vi "GetNetworkTime.vi"(8 "error in (no error)":errorcluster, 11 "NetworkPlugin in":refnum<class "NetworkPlugin.lvclass">) -> (0 "error out":errorcluster, 3 "NetworkPlugin out":refnum<class "NetworkPlugin.lvclass">)   [LabVIEW 2014, in "NetworkImpairmentPlugins.lvlib" / "NetworkPlugin.lvclass"]
uses:
  NetworkPlugin.lvclass
  NetworkImpairmentPluginBase_class/Accessors/Read TimeArray.vi
  NetworkImpairmentPluginBase_class/Accessors/Read NetImpParams.vi
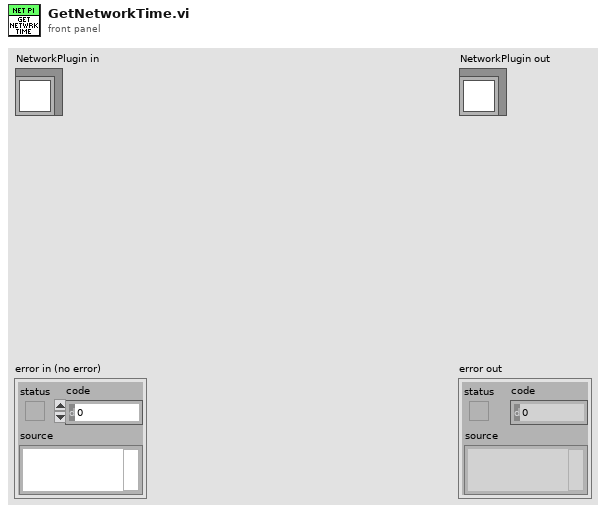
[diagram p1: front panel]
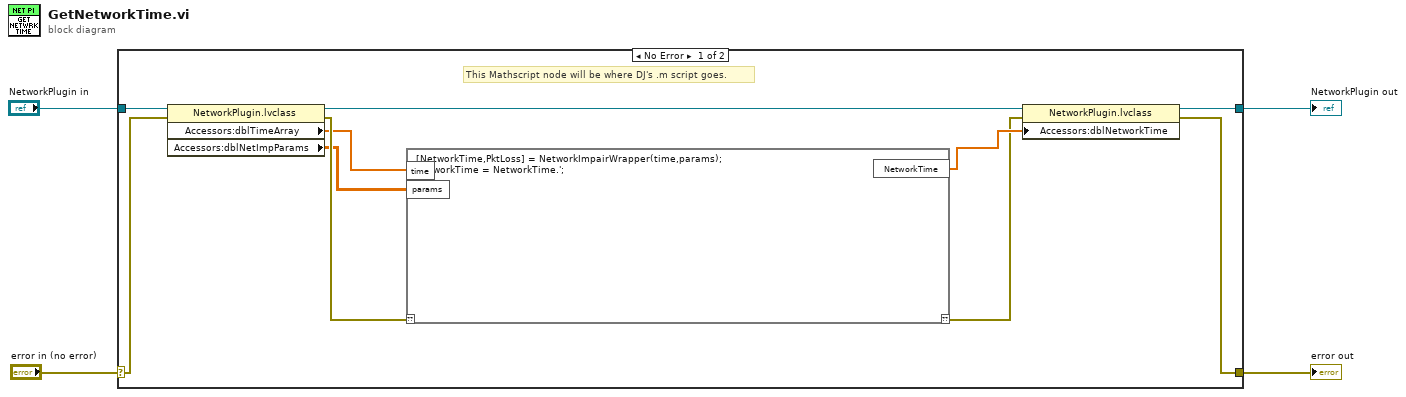
[diagram p0: block diagram]
diagram:
  n1 = case shown="No Error" "error in (no error)" {
    selector: "error in (no error)" -> [w10 w16]
    tunnel: [w9 w16] -> w3
    tunnel: [w13 w15] -> w4
    tunnel: "NetworkPlugin in" -> [w14 w15]
    frame No Error {
      # "This Mathscript node will be where DJ's .m script goes."
      n2 = property class="NetworkPlugin.lvclass"(reference=w14, error in=w10) -> (reference out=w12:refnum<class "NetworkPlugin.lvclass">, error out=w8:errorcluster, "Accessors:dblTimeArray"=w5:dbl[], "Accessors:dblNetImpParams"=w6:dbl[][])
      n3 = script code="[NetworkTime,PktLoss] = NetworkImpairWrapper(time,params);\nNetworkTime = NetworkTime.';"("??"=w8, "time"=w5, "params"=w6) -> ("??"=w7:errorcluster, "NetworkTime"=w11:dbl[])
      n4 = property class="NetworkPlugin.lvclass"(reference=w12, error in=w7, "Accessors:dblNetworkTime"=w11) -> (reference out=w13:refnum<class "NetworkPlugin.lvclass">, error out=w9:errorcluster)
    }
    frame Error {
    }
  }
  "error out" <- w3
  "NetworkPlugin out" <- w4
